vi "Write VI reference.vi"(8 "error in (no error)":errorcluster, 10 "VI reference":refnum<vi>, 11 "UI Load SubPanel Display in":refnum<class "UI Load SubPanel Display.lvclass">) -> (0 "error out":errorcluster, 3 "UI Load SubPanel Display out":refnum<class "UI Load SubPanel Display.lvclass">)   [LabVIEW 2011, in "UI Load SubPanel Display.lvclass"]
uses:
  UI Load SubPanel Display.lvclass
  UI Load SubPanel Display.lvclass/UI Load SubPanel Display.ctl
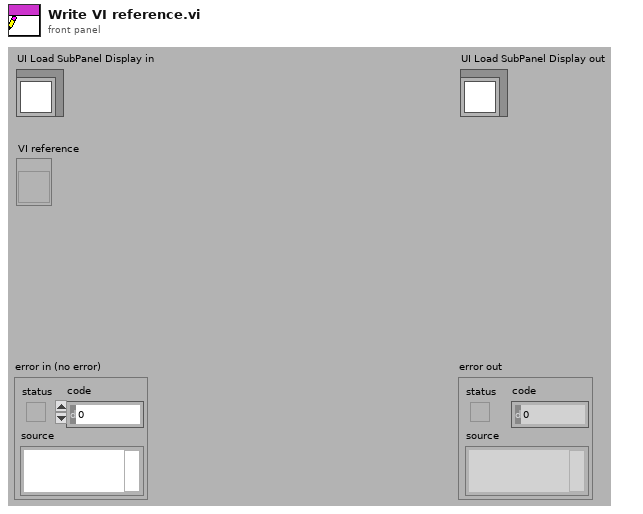
[diagram p1: front panel]
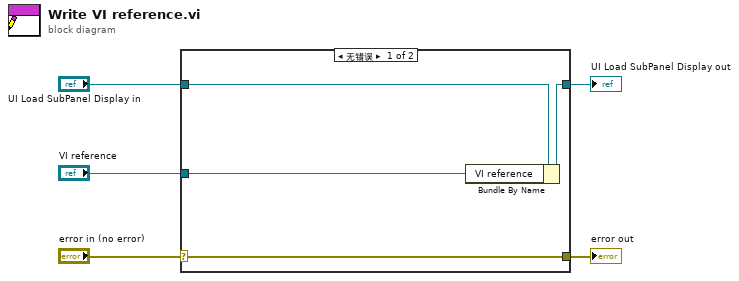
[diagram p0: block diagram]
diagram:
  n1 = case shown="无错误" "error in (no error)" {
    selector: "error in (no error)" -> [w9 w10]
    tunnel: [w9 w10] -> w4
    tunnel: [w7 w11] -> w2
    tunnel: "UI Load SubPanel Display in" -> [w8 w11]
    tunnel: "VI reference" -> [w6 _]
    frame No Error {
      n2 = Bundle By Name(cluster=w8, "VI reference"=w6) -> (w7:refnum<class "UI Load SubPanel Display.lvclass">)
    }
    frame Error {
    }
  }
  "error out" <- w4
  "UI Load SubPanel Display out" <- w2
